vi "Create System Limit Read.vi"(8 "error in (no error)":errorcluster, 11 "Device Item Ref in":T1 format="%.0x") -> (0 "error out":errorcluster)   [LabVIEW 2020, in "G5 Regatron Custom Device System Explorer.lvlib"]
uses:
  G5 Regatron Custom Device System Explorer.lvlib
  <vilib>/NI VeriStand/Custom Device API/Custom Device Channel Type.ctl
  <vilib>/NI VeriStand/Custom Device API/Custom Device API.lvlib
  <vilib>/NI VeriStand/Custom Device API/Custom Device Channel.ctl
  <vilib>/NI VeriStand/Custom Device API/Custom Device Item Ref.ctl
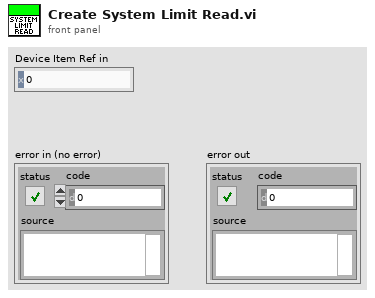
[diagram p1: front panel]
types:
  T1 = typedef "Custom Device API.lvlib/Custom Device Item Ref.ctl" = u64
  T2 = typedef "Custom Device API.lvlib/Custom Device Channel.ctl" = cluster{"Type":T3, "Units":string, "Default Value":dbl, "Faultable":bool, "Scalable":bool}
  T3 = typedef "Custom Device API.lvlib/Custom Device Channel Type.ctl" = enum16{"Input", "Output"}
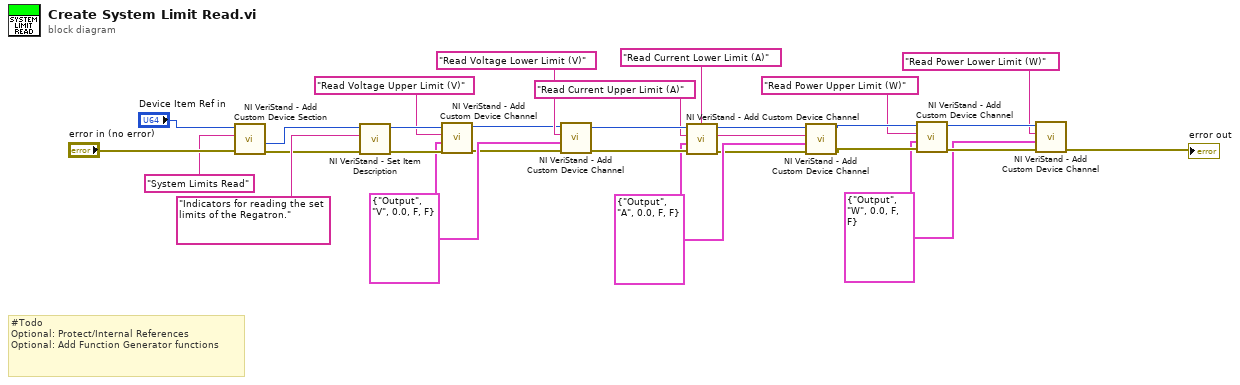
[diagram p0: block diagram]
diagram:
  w14 = T2 {"Type"=enum."Output", "Units"="W", "Default Value"=0.0, "Faultable"=FALSE, "Scalable"=FALSE} ("Channel")
  w11 = T2 {"Type"=enum."Output", "Units"="V", "Default Value"=0.0, "Faultable"=FALSE, "Scalable"=FALSE} ("Channel")
  w5 = T2 {"Type"=enum."Output", "Units"="A", "Default Value"=0.0, "Faultable"=FALSE, "Scalable"=FALSE} ("Channel")
  # "#Todo\nOptional: Protect/Internal References\nOptional: Add Function Generator functions"
  n1 = call <vilib>:"NI VeriStand - Add Custom Device Section.vi"("error in (no error)"="error in (no error)", "Section Name"="System Limits Read", "Parent Ref in"="Device Item Ref in") -> ("error out"=w24:errorcluster, "Section Ptr"=w26:T1)  [unwired: 5 in, 2 out]
  n2 = call <vilib>:"NI VeriStand - Set Item Description.vi"("error in (no error)"=w24, "Description"="Indicators for reading the set limits of the Regatron.", "Item Ref in"=w26) -> ("error out"=w25:errorcluster, "Item Ref out"=w27:T1)  [unwired: 6 in, 1 out]
  n3 = call <vilib>:"NI VeriStand - Add Custom Device Channel.vi"("error in (no error)"=w25, "Channel"=w11, "Channel Name"="Read Voltage Upper Limit (V)", "Parent Ref in"=w27) -> ("error out"=w8:errorcluster, "Parent Ref out"=w9:T1)  [unwired: 4 in, 2 out]
  n4 = call <vilib>:"NI VeriStand - Add Custom Device Channel.vi"("error in (no error)"=w8, "Channel"=w11, "Channel Name"="Read Voltage Lower Limit (V)", "Parent Ref in"=w9) -> ("error out"=w13:errorcluster, "Parent Ref out"=w12:T1)  [unwired: 4 in, 2 out]
  n5 = call <vilib>:"NI VeriStand - Add Custom Device Channel.vi"("error in (no error)"=w13, "Channel"=w5, "Channel Name"="Read Current Upper Limit (A)", "Parent Ref in"=w12) -> ("error out"=w2:errorcluster, "Parent Ref out"=w3:T1)  [unwired: 4 in, 2 out]
  n6 = call <vilib>:"NI VeriStand - Add Custom Device Channel.vi"("error in (no error)"=w2, "Channel"=w5, "Channel Name"="Read Current Lower Limit (A)", "Parent Ref in"=w3) -> ("error out"=w20:errorcluster, "Parent Ref out"=w19:T1)  [unwired: 4 in, 2 out]
  n7 = call <vilib>:"NI VeriStand - Add Custom Device Channel.vi"("error in (no error)"=w20, "Channel"=w14, "Channel Name"="Read Power Upper Limit (W)", "Parent Ref in"=w19) -> ("error out"=w17:errorcluster, "Parent Ref out"=w16:T1)  [unwired: 4 in, 2 out]
  n8 = call <vilib>:"NI VeriStand - Add Custom Device Channel.vi"("error in (no error)"=w17, "Channel"=w14, "Channel Name"="Read Power Lower Limit (W)", "Parent Ref in"=w16) -> ("error out"=→"error out":errorcluster)  [unwired: 4 in, 3 out]
